vi "logon.vi"(6 "Display error messages?":bool=TRUE, 8 "error in":errorcluster, 10 "data server address in":string, 11 "port":u16=6341) -> (0 "error out":errorcluster, 1 "Server stats":T1={"scan rate"=10.0, "# connections"=0, "channel settings"=[]} {"channel settings"."lower input limits" format="%.4f"; "channel settings"."upper input limits" format="%.4f"; "scan rate" format="%.2f"}, 2 "data server address":string="128.84.245.227", 3 "connection ID":refnum<k5>)   [LabVIEW 2012]
doc: "Open data server opens a connection with a data server. If the array of data servers contains only one element then the connection is made immediately. If the array contains more than one element a subvi with a dialog box opens to select the data server. TCP is then used to log on to the data server and data server information is returned in the Server Stats control.\n\nInputs\n\nPort - TCP port number. Must be the same as the port number used by the data server. At Cornell CEE we use port 6341.\n\nData Servers - An array of strings that are either names or IP addresses for available dataservers \n\nError in - \n\nOutputs\n\nData server address - String containing the name or the IP address of the selected data server.\n\nRestart - Boolean that is true if the connection with the data server could not be established.\n\nServer Stats - Data server information including scan rate, number of client connections and channel information.\n\nError out - \n\n\nCreated by Monroe Weber-Shirk\nCornell University\nmw24@cornell.edu\nJanuary 2000"
uses:
  DataServer/Server stats.ctl
  DataServer/Server Stats.vi
panel:
  # "Hz"
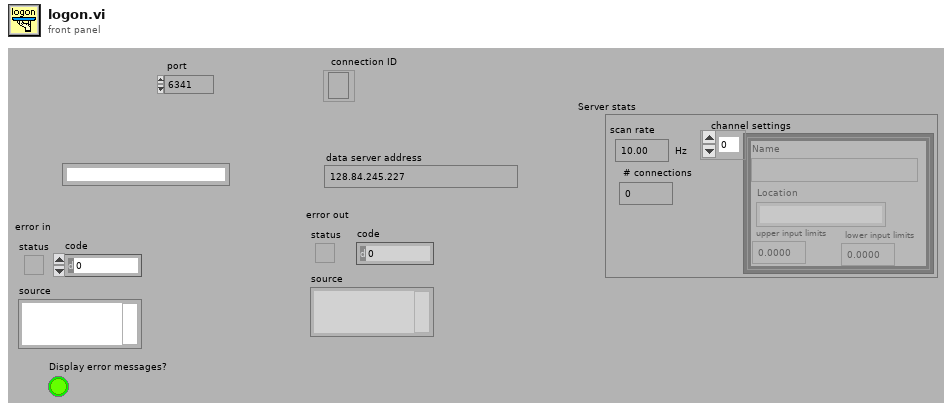
[diagram p1: front panel]
types:
  T1 = typedef "Server stats.ctl" = cluster{"scan rate":dbl, "# connections":i32, "channel settings":cluster{"Name":string, "upper input limits":sgl, "lower input limits":sgl, "Location":string}[]}
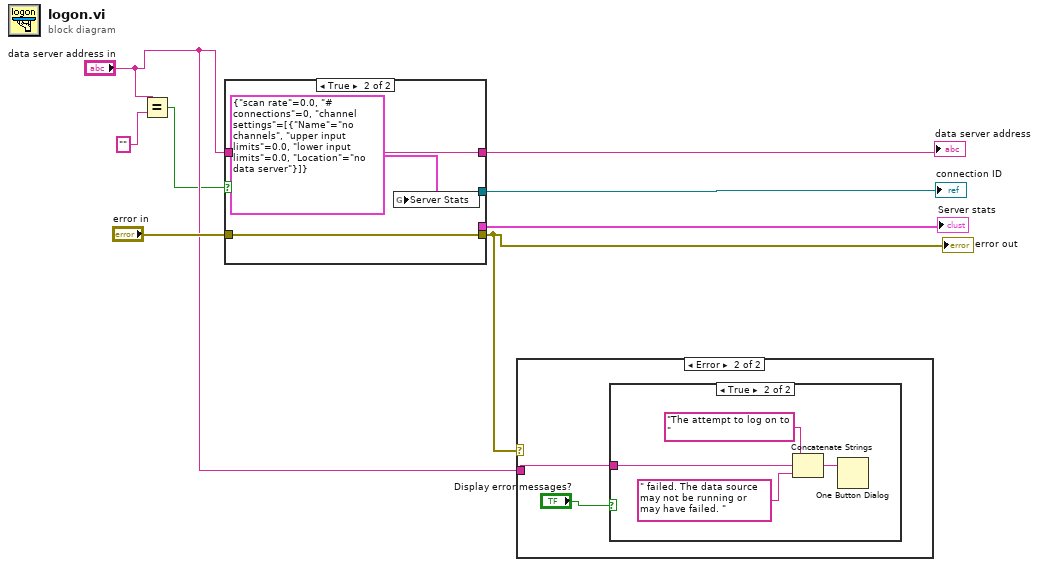
[diagram p0: block diagram]
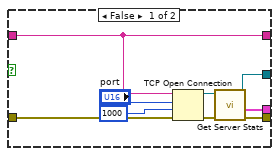
[diagram p2: hidden frame]
diagram:
  n1 = Equal?(x="data server address in", y="") -> (x = y?=w1:bool)
  n2 = case shown="True" w1 {
    tunnel: [w17 _] -> w8
    tunnel: "error in" -> [w16 w20]
    tunnel: [w15 _] -> w6
    tunnel: [w10 w20] -> w5
    tunnel: "data server address in" -> [w9 w19]
    tunnel: [w9 w19] -> w4
    frame False {
      n3 = TCP Open Connection(address=w9, remote port or service name="port", timeout ms (60000)=1000, error in (no error)=w16) -> (connection ID=w12:refnum<k5>, error out=w13:errorcluster)  [unwired: 1 in]
      n4 = call "Get Server Stats.vi"("error in (no error)"=w13, "Connection ID"=w12) -> ("error out"=w10:errorcluster, "Server stats"=w15:T1, "Connection ID"=w17:refnum<k5>)  [unwired: 6 in, 1 out]
    }
    frame True {
      n5 = global write "Server Stats.vi" "Server Stats"(T1 {"scan rate"=0.0, "# connections"=0, "channel settings"=[{"Name"="no channels", "upper input limits"=0.0, "lower input limits"=0.0, "Location"="no data server"}]} ("Server Stats")) -> ()
    }
  }
  "data server address" <- w4
  "connection ID" <- w8
  "error out" <- w5
  "Server stats" <- w6
  n6 = case shown="Error" w5 {
    tunnel: "data server address in" -> [_ w22]
    frame No Error {
    }
    frame Error {
      n7 = case shown="True" "Display error messages?" {
        tunnel: w22 -> [_ w24]
        frame False {
        }
        frame True {
          n8 = Concatenate Strings("The attempt to log on to  " ("message"), w24, " failed. The data source may not be running or may have failed. " ("message")) -> (w23:string)
          n9 = One Button Dialog(message=w23) -> ()  [unwired: 1 in, 1 out]
        }
      }
    }
  }
